vi "Close All Notifier.vi"(8 "error in (no error)":errorcluster, 11 "All Display Notifiers In":T1) -> (0 "error out":errorcluster)   [LabVIEW 2014]
uses:
  All Display Notifiers.ctl
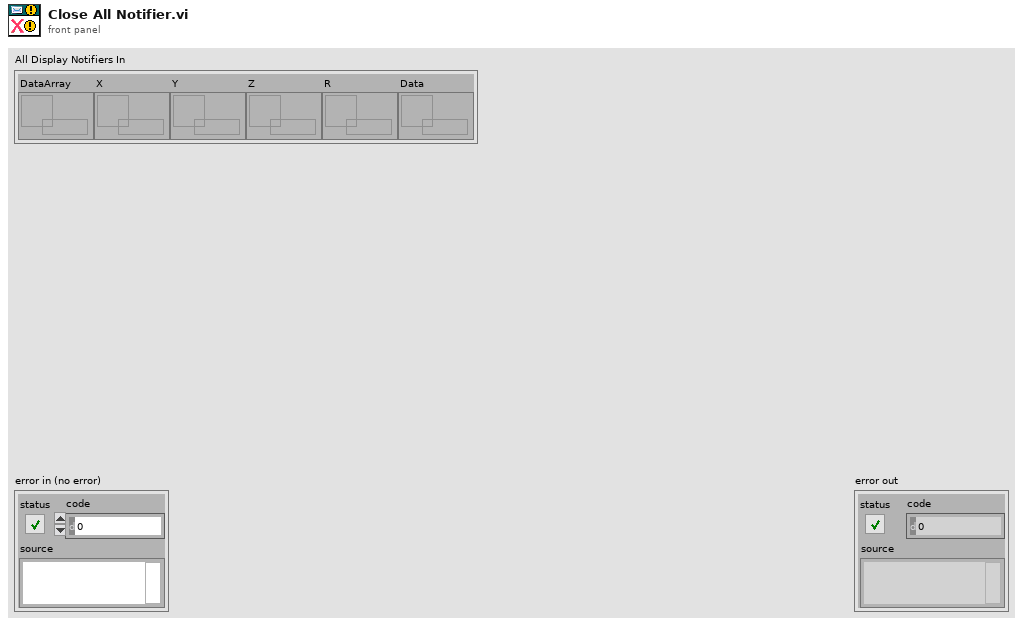
[diagram p1: front panel]
types:
  T1 = typedef "All Display Notifiers.ctl" = cluster{"DataArray":refnum<queue>, "X":refnum<queue>, "Y":refnum<queue>, "Z":refnum<queue>, "R":refnum<queue>, "Data":refnum<queue>}
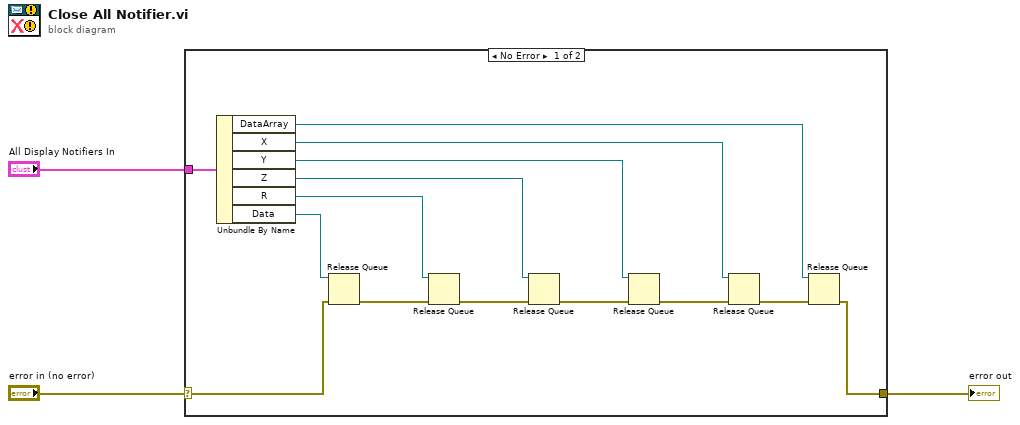
[diagram p0: block diagram]
diagram:
  n1 = case shown="No Error" "error in (no error)" {
    selector: "error in (no error)" -> [w11 w18]
    tunnel: "All Display Notifiers In" -> [w17 _]
    tunnel: [w4 w18] -> w1
    frame No Error {
      n2 = Unbundle By Name(w17) -> ("DataArray"=w5:refnum<queue>, "X"=w12:refnum<queue>, "Y"=w13:refnum<queue>, "Z"=w14:refnum<queue>, "R"=w15:refnum<queue>, "Data"=w16:refnum<queue>)
      n3 = Release Queue(queue=w16, error in (no error)=w11) -> (error out=w10:errorcluster)  [unwired: 1 in, 2 out]
      n4 = Release Queue(queue=w15, error in (no error)=w10) -> (error out=w9:errorcluster)  [unwired: 1 in, 2 out]
      n5 = Release Queue(queue=w14, error in (no error)=w9) -> (error out=w8:errorcluster)  [unwired: 1 in, 2 out]
      n6 = Release Queue(queue=w13, error in (no error)=w8) -> (error out=w7:errorcluster)  [unwired: 1 in, 2 out]
      n7 = Release Queue(queue=w12, error in (no error)=w7) -> (error out=w6:errorcluster)  [unwired: 1 in, 2 out]
      n8 = Release Queue(queue=w5, error in (no error)=w6) -> (error out=w4:errorcluster)  [unwired: 1 in, 2 out]
    }
    frame Error {
    }
  }
  "error out" <- w1
